vi "Initialize.vi"(7 "timeout, ms (1000)":u32=1000, 8 "error in (no error)":errorcluster, 10 "baud rate (38400)":u32=38400, 11 "port":refnum<visa-resource-name>) -> (0 "error out":errorcluster, 3 "ProPar out":refnum<class "PL Bronkhorst ProPar.lvclass">)   [LabVIEW 2015, in "PL Bronkhorst ProPar.lvclass"]
doc: "Initializes connection to device using specified settings."
uses:
  PL Bronkhorst ProPar.lvclass
  PL Bronkhorst ProPar.lvclass/PL Bronkhorst ProPar.ctl
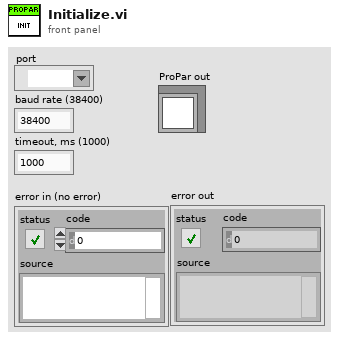
[diagram p1: front panel]
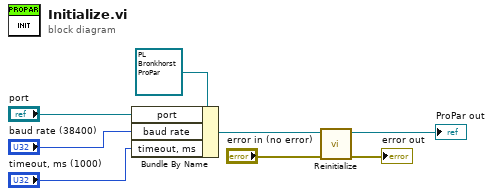
[diagram p0: block diagram]
diagram:
  n1 = Bundle By Name(cluster=refnum<class "PL Bronkhorst ProPar.lvclass"> refnum ("PL Comdel CX.lvclass"), "port"="port", "baud rate"="baud rate (38400)", "timeout, ms"="timeout, ms (1000)") -> (w8:refnum<class "PL Bronkhorst ProPar.lvclass">)
  n2 = call "Reinitialize.vi"("error in (no error)"="error in (no error)", "ProPar in"=w8) -> ("error out"=→"error out":errorcluster, "ProPar out"=→"ProPar out":refnum<class "PL Bronkhorst ProPar.lvclass">)  [unwired: 8 in]
